vi "AFG3022_Arb_Fun_Control.vi"(10 "Channel":u16(ring) items=["Channel 1", "Channel 2"], 11 "Function Selector":u16(ring) items=["Sine", "Square", "Ramp", "Assymetric Sine", "Assymetric Arbitrary"]) -> ()   [LabVIEW 2012]
uses:
  ADAM Client/Sub VIs/ADAM Controls/Update_scan_value.ctl
panel:
  in  "Amp Gain":dbl=73.0
  in  "AM?":bool
  in  "Deviation Frequency":dbl=500.0
  in  "Modulation Frequency":dbl=20.0
  in  "FM?":bool
  in  "Channel 2 Phase":dbl
  in  "Channel 1 Phase":dbl
  in  "Set Zero Mean":bool
  out "Amplitude":dbl=120.0
  in  "Set Amplitude":bool
  out "Ts/T":dbl=0.32
  in  "Time Ratio":dbl[](array[slide])=[0.07, 0.15, 0.1, 0.6799999999999999] min=0.0 max=1.0 step=0.01 scale=0.0..1.0
  in  "Fine Amp":dbl(knob) min=0.0 max=1.0 step=0.1 scale=0.0..1.0
  in  "Course Amp":dbl(knob)=120.0 min=0.0 max=120.0 step=2.0 scale=0.0..120.0
  in  "Channel 2":bool
  in  "Channel 1":bool
  in  "Set Frequency":bool
  in  "Scale":u16(ring)=2 items=["1", "10", "100", "1k", "10k"]
  in  "Fine Freq":dbl(knob)=0.5 min=0.0 max=1.0 step=0.1 scale=0.0..1.0
  in  "Course Freq":dbl(knob)=9.0 min=0.0 max=10.0 step=1.0 scale=0.0..10.0
  in  "Stop Button":bool
  in  "VISA resource name":refnum<visa-resource-name>="USB0::0x0699::0x0347::C036837::INSTR"
  out "Frequency":dbl=950.0
  # "Suction Time"
  # "Blowing Time"
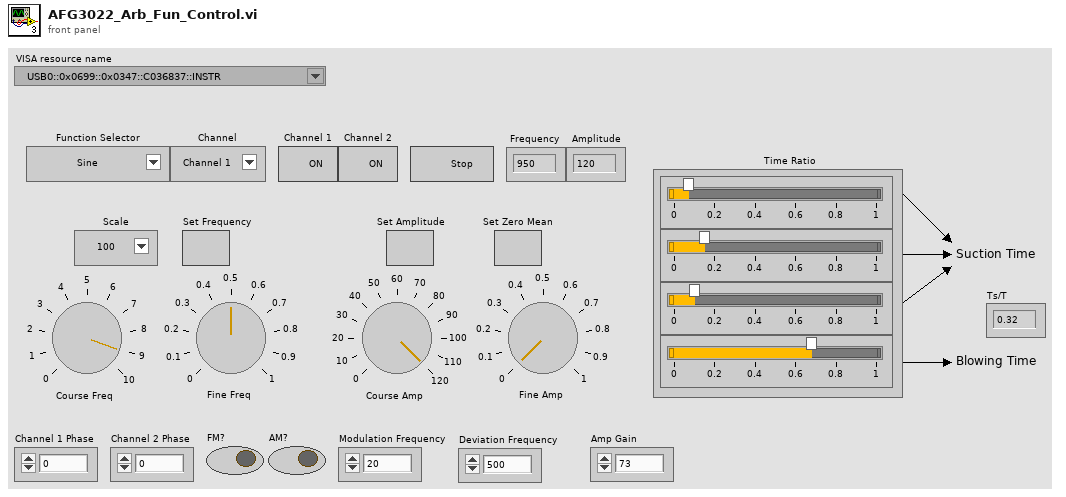
[diagram p1: front panel]
types:
  T1 = typedef "Update_scan_value.ctl" = cluster{"Channel Name":string, "New Value":dbl}
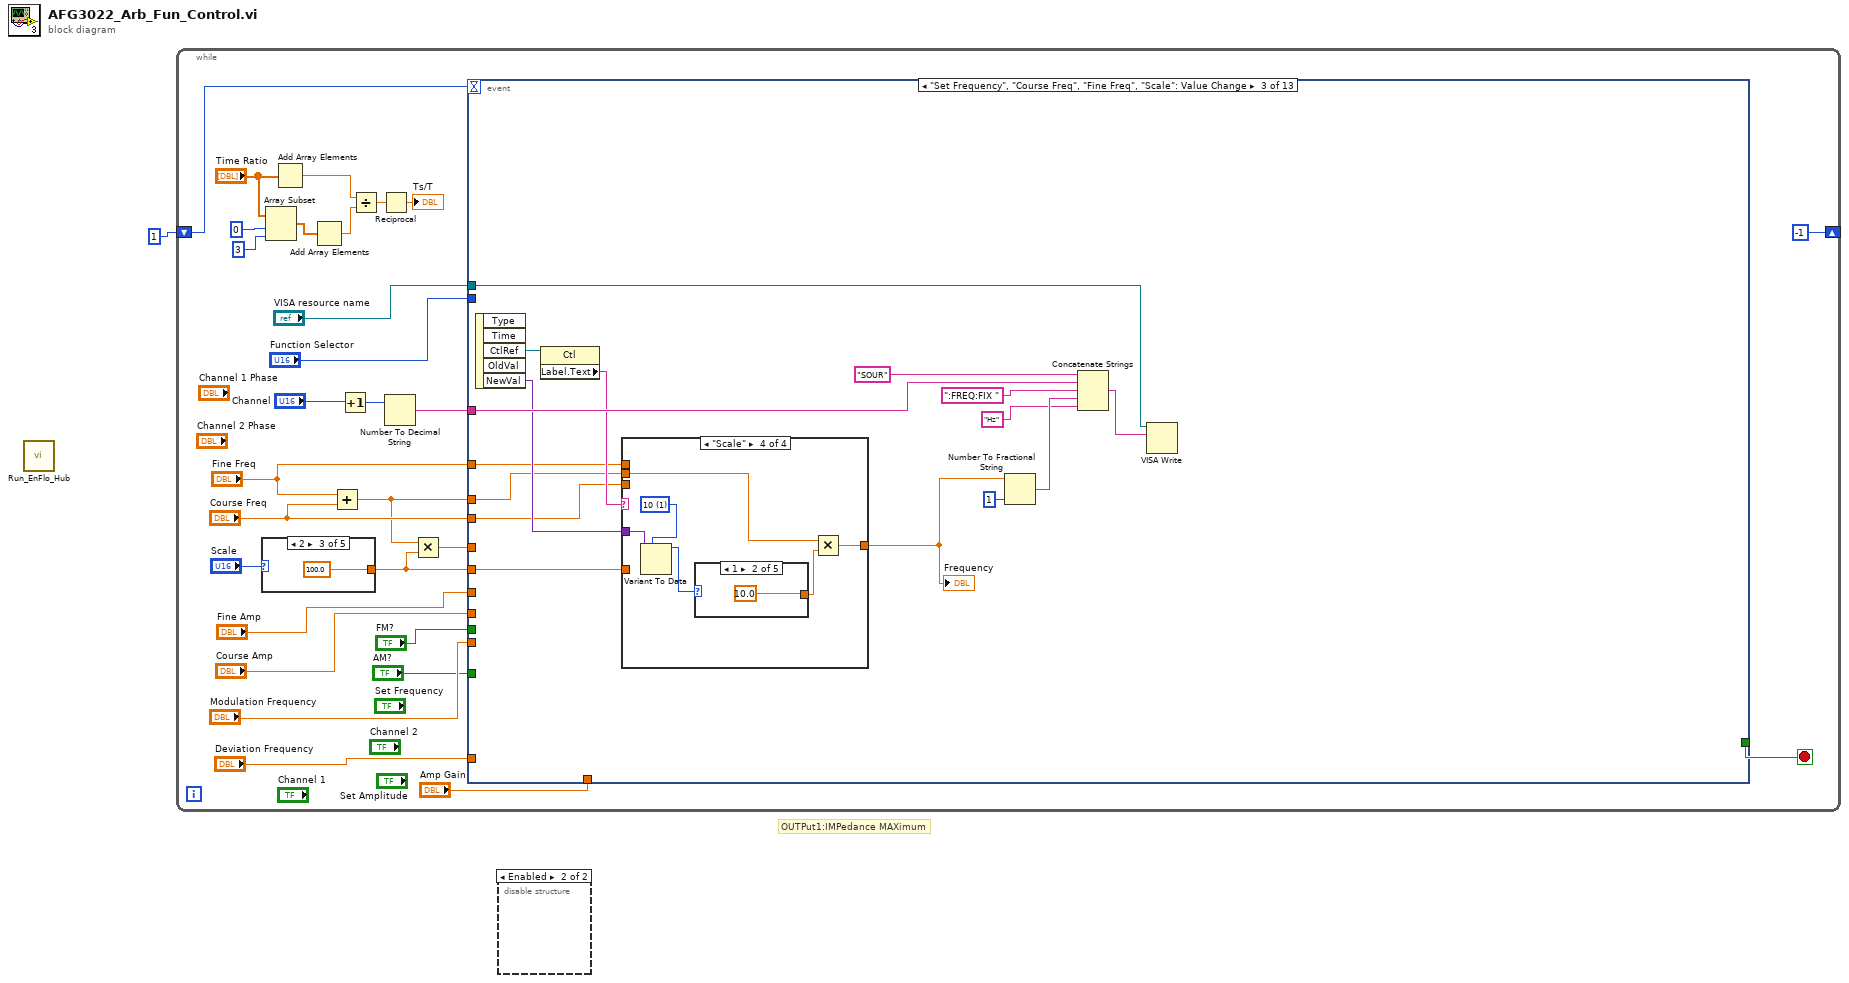
[diagram p0: block diagram]
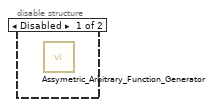
[diagram p2: hidden frame]
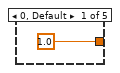
[diagram p3: hidden frame]
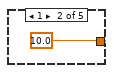
[diagram p4: hidden frame]
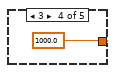
[diagram p5: hidden frame]
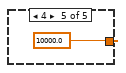
[diagram p6: hidden frame]
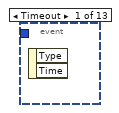
[diagram p7: hidden frame]
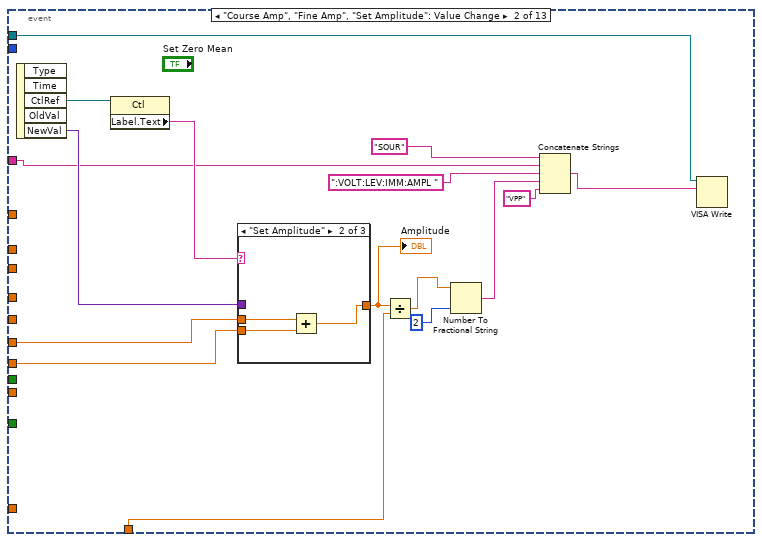
[diagram p8: hidden frame]
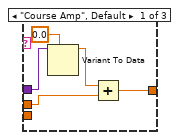
[diagram p9: hidden frame]
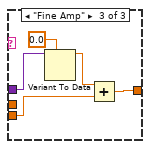
[diagram p10: hidden frame]
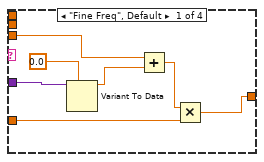
[diagram p11: hidden frame]
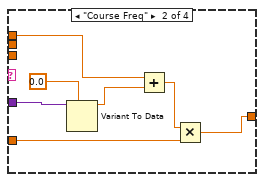
[diagram p12: hidden frame]
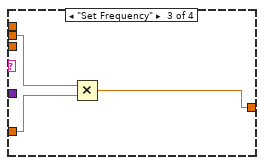
[diagram p13: hidden frame]
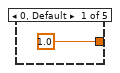
[diagram p14: hidden frame]
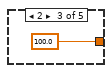
[diagram p15: hidden frame]
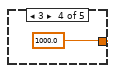
[diagram p16: hidden frame]
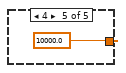
[diagram p17: hidden frame]
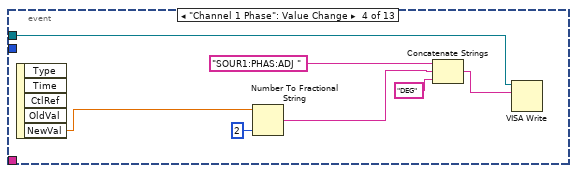
[diagram p18: hidden frame]
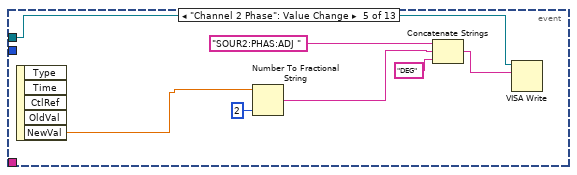
[diagram p19: hidden frame]
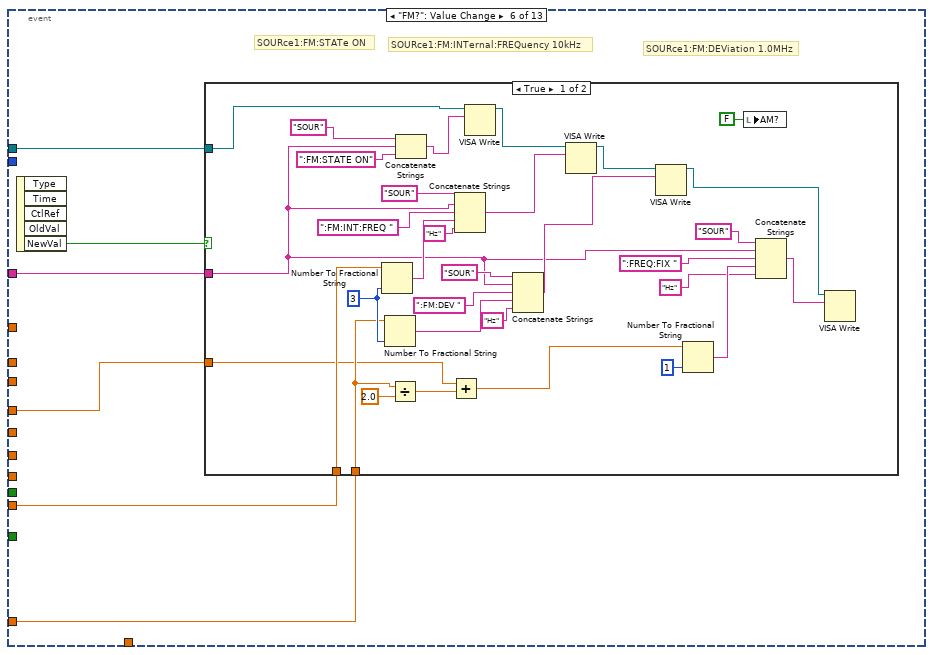
[diagram p20: hidden frame]
diagram:
  # "OUTPut1:IMPedance MAXimum"
  n1 = call "Run_EnFlo_Hub.vi"() -> ()  [unwired: 8 in]
  n2 = while {
    shift-right: [-1] -> _
    shift-left: 1 -> [w27]
    stop <- w29 stop-if-true
    n3 = case shown="2" "Scale" {
      tunnel: [1.0 10.0 100.0 1000.0 10000.0] -> w6
      frame 0, Default {
      }
      frame 1 {
      }
      frame 2 {
      }
      frame 3 {
      }
      frame 4 {
      }
    }
    n4 = Array Subset(array="Time Ratio", index=0, length=3) -> (w15:dbl[])
    n5 = Add Array Elements(numeric array="Time Ratio") -> (sum=w14:dbl)
    n6 = Add Array Elements(numeric array=w15) -> (sum=w13:dbl)
    n7 = Add(x="Fine Freq", y="Course Freq") -> (x+y=w5:dbl)
    n8 = Increment(x="Channel") -> (x+1=w25:u16)
    n9 = Divide(x=w14, y=w13) -> (x/y=w12:dbl)
    n10 = Reciprocal(x=w12) -> (1/x=→"Ts/T":dbl)
    n11 = Number To Decimal String(number=w25) -> (decimal integer string=w23:string)  [unwired: 1 in]
    n12 = Multiply(x=w5, y=w6) -> (x*y=w4:dbl)
    n13 = event shown="[2] \"Set Frequency\", \"Course Freq\", \"Fine Freq\", \"Scale\": Value Change" {
      selector: _ -> [_ _ _ _ _ _ _ _ _ _ _ _ _]
      dyn-events: _ -> [_ _ _ _ _ _ _ _ _ _ _ _ _]
      timeout: w27 -> [_ _ _ _ _ _ _ _ _ _ _ _ _]
      tunnel: "VISA resource name" -> [_ w39 w75 w113 w117 w126 w177 w220 w236 w265 w277 w309 _]
      tunnel: [_ _ _ _ _ _ _ _ _ _ _ _ "Stop Button"] -> w29
      tunnel: w23 -> [_ w40 w73 _ _ w127 w176 w219 w235 _ _ w288 _]
      tunnel: w5 -> [_ _ w69 _ _ _ _ _ _ _ _ _ _]
      tunnel: "Course Freq" -> [_ _ w67 _ _ _ _ _ _ _ _ _ _]
      tunnel: w6 -> [_ _ w66 _ _ _ _ _ _ _ _ _ _]
      tunnel: "Fine Freq" -> [_ _ w65 _ _ _ _ _ _ _ _ _ _]
      tunnel: "Course Amp" -> [_ w48 _ _ _ _ _ _ _ _ _ w289 _]
      tunnel: "Fine Amp" -> [_ w47 _ _ _ _ _ _ _ _ _ w290 _]
      tunnel: "Function Selector" -> [_ _ _ _ _ _ _ _ _ _ _ w286 _]
      tunnel: "Modulation Frequency" -> [_ _ _ _ _ w125 w175 _ _ _ _ _ _]
      tunnel: "FM?" -> [_ _ _ _ _ _ _ w215 w237 _ _ _ _]
      tunnel: "Deviation Frequency" -> [_ _ _ _ _ w124 _ _ _ _ _ _ _]
      tunnel: w4 -> [_ _ _ _ _ w123 w174 _ w233 _ _ _ _]
      tunnel: "AM?" -> [_ _ _ _ _ _ _ w217 _ _ _ _ _]
      tunnel: "Amp Gain" -> [_ w37 _ _ _ _ _ _ _ _ _ w282 _]
      event Timeout {
        n14 = event-data() -> ()  [unwired: 1 in, 2 out]
      }
      event "Course Amp", "Fine Amp", "Set Amplitude": Value Change {
        n15 = event-data() -> ("CtlRef"=w51:refnum<vi>, "NewVal"=w49:variant)  [unwired: 1 in, 3 out]
        n16 = property class="Ctl"(reference=w51) -> ("Label.Text"=w50:string)  [unwired: 1 in, 2 out]
        n17 = case shown="\"Set Amplitude\"" w50 {
          tunnel: w49 -> [w53 _ w61]
          tunnel: w48 -> [_ w58 w64]
          tunnel: w47 -> [w56 w59 _]
          tunnel: [w55 w57 w63] -> w36
          frame "Course Amp", Default {
            n18 = Variant To Data(type=0.0 ("Fine Amp"), Variant=w53) -> (data=w52:dbl)  [unwired: 1 in, 1 out]
            n19 = Add(x=w52, y=w56) -> (x+y=w55:dbl)
          }
          frame "Set Amplitude" {
            n20 = Add(x=w59, y=w58) -> (x+y=w57:dbl)
          }
          frame "Fine Amp" {
            n21 = Variant To Data(type=0.0 ("Fine Amp"), Variant=w61) -> (data=w60:dbl)  [unwired: 1 in, 1 out]
            n22 = Add(x=w60, y=w64) -> (x+y=w63:dbl)
          }
        }
        "Amplitude" <- w36
        n23 = Divide(x=w36, y=w37) -> (x/y=w38:dbl)
        n24 = Number To Fractional String(number=w38, precision (6)=i16 2) -> (F-format string=w42:string)  [unwired: 2 in]
        n25 = Concatenate Strings("SOUR" ("string"), w40, ":VOLT:LEV:IMM:AMPL " ("string"), w42, "VPP" ("string")) -> (w43:string)
        n26 = VISA Write(VISA resource name=w39, write buffer=w43) -> ()  [unwired: 1 in, 3 out]
      }
      event "Set Frequency", "Course Freq", "Fine Freq", "Scale": Value Change {
        n27 = event-data() -> ("CtlRef"=w72:refnum<vi>, "NewVal"=w70:variant)  [unwired: 1 in, 3 out]
        n28 = property class="Ctl"(reference=w72) -> ("Label.Text"=w71:string)  [unwired: 1 in, 2 out]
        n29 = case shown="\"Scale\"" w71 {
          tunnel: w70 -> [w87 w94 _ w103]
          tunnel: w69 -> [_ _ w97 w99]
          tunnel: [w81 w88 w95 w98] -> w68
          tunnel: w67 -> [w84 _ _ _]
          tunnel: w66 -> [w82 w90 w96 _]
          tunnel: w65 -> [_ w89 _ _]
          frame "Fine Freq", Default {
            n30 = Variant To Data(type=0.0, Variant=w87) -> (data=w85:dbl)  [unwired: 1 in, 1 out]
            n31 = Add(x=w84, y=w85) -> (x+y=w83:dbl)
            n32 = Multiply(x=w83, y=w82) -> (x*y=w81:dbl)
          }
          frame "Course Freq" {
            n33 = Variant To Data(type=0.0, Variant=w94) -> (data=w92:dbl)  [unwired: 1 in, 1 out]
            n34 = Add(x=w89, y=w92) -> (x+y=w91:dbl)
            n35 = Multiply(x=w91, y=w90) -> (x*y=w88:dbl)
          }
          frame "Set Frequency" {
            n36 = Multiply(x=w97, y=w96) -> (x*y=w95:dbl)
          }
          frame "Scale" {
            w102 = u16 1 items=["1", "10", "100", "1k", "10k"] ("Scale")
            n37 = Variant To Data(type=w102, Variant=w103) -> (data=w101:u16)  [unwired: 1 in, 1 out]
            n38 = case shown="1" w101 {
              tunnel: [1.0 10.0 100.0 1000.0 10000.0] -> w100
              frame 0, Default {
              }
              frame 1 {
              }
              frame 2 {
              }
              frame 3 {
              }
              frame 4 {
              }
            }
            n39 = Multiply(x=w99, y=w100) -> (x*y=w98:dbl)
          }
        }
        "Frequency" <- w68
        n40 = Number To Fractional String(number=w68, precision (6)=i16 1) -> (F-format string=w77:string)  [unwired: 2 in]
        n41 = Concatenate Strings("SOUR", w73, ":FREQ:FIX " ("string"), w77, "Hz" ("string")) -> (w74:string)
        n42 = VISA Write(VISA resource name=w75, write buffer=w74) -> ()  [unwired: 1 in, 3 out]
      }
      event "Channel 1 Phase": Value Change {
        n43 = event-data() -> ("NewVal"=w112:dbl)  [unwired: 1 in, 4 out]
        n44 = Number To Fractional String(number=w112, precision (6)=i16 2) -> (F-format string=w110:string)  [unwired: 2 in]
        n45 = Concatenate Strings("SOUR1:PHAS:ADJ ", w110, "DEG" ("string")) -> (w114:string)
        n46 = VISA Write(VISA resource name=w113, write buffer=w114) -> ()  [unwired: 1 in, 3 out]
      }
      event "Channel 2 Phase": Value Change {
        n47 = event-data() -> ("NewVal"=w116:dbl)  [unwired: 1 in, 4 out]
        n48 = Number To Fractional String(number=w116, precision (6)=i16 2) -> (F-format string=w119:string)  [unwired: 2 in]
        n49 = Concatenate Strings("SOUR2:PHAS:ADJ ", w119, "DEG" ("string")) -> (w121:string)
        n50 = VISA Write(VISA resource name=w117, write buffer=w121) -> ()  [unwired: 1 in, 3 out]
      }
      event "FM?": Value Change {
        # "SOURce1:FM:DEViation 1.0MHz"
        # "SOURce1:FM:INTernal:FREQuency 10kHz"
        # "SOURce1:FM:STATe ON"
        n51 = event-data() -> ("NewVal"=w128:bool)  [unwired: 1 in, 4 out]
        n52 = case shown="True" w128 {
          tunnel: w127 -> [w131 w162]
          tunnel: w126 -> [w158 w171]
          tunnel: w125 -> [w152 _]
          tunnel: w124 -> [w144 _]
          tunnel: w123 -> [w142 w161]
          frame True {
            w149 = i16 3 ("precision (6)")
            n53 = Number To Fractional String(number=w152, precision (6)=w149) -> (F-format string=w151:string)  [unwired: 2 in]
            n54 = Number To Fractional String(number=w144, precision (6)=w149) -> (F-format string=w146:string)  [unwired: 2 in]
            n55 = Divide(x=w144, y=2.0) -> (x/y=w141:dbl)
            n56 = Concatenate Strings("SOUR", w131, ":FM:STATE ON" ("string")) -> (w157:string)
            n57 = Add(x=w142, y=w141) -> (x+y=w130:dbl)
            n58 = Concatenate Strings("SOUR", w131, ":FM:INT:FREQ " ("string"), w151, "Hz" ("string")) -> (w153:string)
            n59 = VISA Write(VISA resource name=w158, write buffer=w157) -> (VISA resource name out=w156:refnum<visa-resource-name>)  [unwired: 1 in, 2 out]
            n60 = Concatenate Strings("SOUR", w131, ":FM:DEV " ("string"), w146, "Hz" ("string")) -> (w134:string)
            n61 = VISA Write(VISA resource name=w156, write buffer=w153) -> (VISA resource name out=w133:refnum<visa-resource-name>)  [unwired: 1 in, 2 out]
            n62 = VISA Write(VISA resource name=w133, write buffer=w134) -> (VISA resource name out=w132:refnum<visa-resource-name>)  [unwired: 1 in, 2 out]
            n63 = Number To Fractional String(number=w130, precision (6)=i16 1) -> (F-format string=w137:string)  [unwired: 2 in]
            n64 = local write "AM?"(FALSE ("AM?")) -> ()
            n65 = Concatenate Strings("SOUR", w131, ":FREQ:FIX " ("string"), w137, "Hz" ("string")) -> (w135:string)
            n66 = VISA Write(VISA resource name=w132, write buffer=w135) -> ()  [unwired: 1 in, 3 out]
          }
          frame False {
            n67 = Concatenate Strings("SOUR", w162, ":FM:STATE OFF" ("string")) -> (w170:string)
            n68 = VISA Write(VISA resource name=w171, write buffer=w170) -> (VISA resource name out=w163:refnum<visa-resource-name>)  [unwired: 1 in, 2 out]
            n69 = Number To Fractional String(number=w161, precision (6)=i16 1) -> (F-format string=w166:string)  [unwired: 2 in]
            n70 = Concatenate Strings("SOUR", w162, ":FREQ:FIX " ("string"), w166, "Hz" ("string")) -> (w164:string)
            n71 = VISA Write(VISA resource name=w163, write buffer=w164) -> ()  [unwired: 1 in, 3 out]
          }
        }
      }
      event "AM?": Value Change {
        n72 = event-data() -> ("NewVal"=w178:bool)  [unwired: 1 in, 4 out]
        n73 = case shown="True" w178 {
          tunnel: w177 -> [w180 w193]
          tunnel: w176 -> [w179 w209]
          tunnel: w175 -> [_ w200]
          tunnel: w174 -> [_ w185]
          frame False {
            # "SOURce1:AM:STATe OFF"
            n74 = Concatenate Strings("SOUR" ("string"), w179) -> (w181:string)
            n75 = Concatenate Strings(w181, ":AM:STAT OFF" ("string")) -> (w182:string)
            n76 = VISA Write(VISA resource name=w180, write buffer=w182) -> ()  [unwired: 1 in, 3 out]
          }
          frame True {
            # "SOURce1:AM:STATe OFF"
            # "SOURce1:AM:INTernal:FUNCtion SQUare"
            # "SOURce1:AM:INTernal:FREQuency XXHz"
            # "SOURce1:AM:DEPth 100"
            n77 = Number To Fractional String(number=w185, precision (6)=i16 3) -> (F-format string=w188:string)  [unwired: 2 in]
            n78 = Number To Fractional String(number=w200, precision (6)=i16 3) -> (F-format string=w197:string)  [unwired: 2 in]
            n79 = Concatenate Strings("SOUR" ("string"), w209) -> (w191:string)
            n80 = Concatenate Strings(w191, ":AM:INT:FREQ " ("string"), w197, "Hz" ("string")) -> (w199:string)
            n81 = Concatenate Strings(w191, ":AM:STAT ON" ("string")) -> (w207:string)
            n82 = Concatenate Strings(w191, ":AM:DEPT 100" ("string")) -> (w205:string)
            n83 = Concatenate Strings(w191, ":AM:INT:FUNC SQU" ("string")) -> (w194:string)
            n84 = Concatenate Strings(w191, ":FREQ:FIX " ("string"), w188, "Hz" ("string")) -> (w190:string)
            n85 = VISA Write(VISA resource name=w193, write buffer=w190) -> (VISA resource name out=w192:refnum<visa-resource-name>)  [unwired: 1 in, 2 out]
            n86 = VISA Write(VISA resource name=w192, write buffer=w207) -> (VISA resource name out=w211:refnum<visa-resource-name>, error out=w204:errorcluster)  [unwired: 1 in, 1 out]
            n87 = VISA Write(VISA resource name=w211, write buffer=w205, error in (no error)=w204) -> (VISA resource name out=w213:refnum<visa-resource-name>, error out=w203:errorcluster)  [unwired: 1 out]
            n88 = VISA Write(VISA resource name=w213, write buffer=w199, error in (no error)=w203) -> (VISA resource name out=w212:refnum<visa-resource-name>, error out=w202:errorcluster)  [unwired: 1 out]
            n89 = VISA Write(VISA resource name=w212, write buffer=w194, error in (no error)=w202) -> ()  [unwired: 3 out]
            n90 = local write "FM?"(FALSE ("AM?")) -> ()
          }
        }
      }
      event "Modulation Frequency": Value Change {
        n91 = event-data() -> ("NewVal"=w218:dbl)  [unwired: 1 in, 4 out]
        n92 = Or(x=w215, y=w217) -> (x .or. y?=w216:bool)
        n93 = case shown="True" w216 {
          tunnel: w220 -> [_ w225]
          tunnel: w219 -> [_ w224]
          tunnel: w218 -> [_ w223]
          tunnel: w215 -> [_ w221]
          frame False {
          }
          frame True {
            # ":AM:INT:FREQ"
            n94 = case shown="False" w221 {
              tunnel: [":AM:INT:FREQ " ("string") ":FM:INT:FREQ " ("string")] -> w229
              frame False {
              }
              frame True {
              }
            }
            n95 = Number To Fractional String(number=w223, precision (6)=i16 3) -> (F-format string=w227:string)  [unwired: 2 in]
            n96 = Concatenate Strings("SOUR", w224, w229, w227, "Hz" ("string")) -> (w222:string)
            n97 = VISA Write(VISA resource name=w225, write buffer=w222) -> ()  [unwired: 1 in, 3 out]
          }
        }
      }
      event "Deviation Frequency": Value Change {
        n98 = event-data() -> ("NewVal"=w234:dbl)  [unwired: 1 in, 4 out]
        n99 = case shown="True" w237 {
          tunnel: w236 -> [_ w243]
          tunnel: w235 -> [_ w241]
          tunnel: w234 -> [_ w239]
          tunnel: w233 -> [_ w238]
          frame False {
          }
          frame True {
            n100 = Number To Fractional String(number=w239, precision (6)=i16 3) -> (F-format string=w254:string)  [unwired: 2 in]
            n101 = Divide(x=w239, y=2.0) -> (x/y=w251:dbl)
            n102 = Add(x=w238, y=w251) -> (x+y=w244:dbl)
            n103 = Concatenate Strings("SOUR", w241, ":FM:DEV: " ("string"), w254, "Hz" ("string")) -> (w242:string)
            n104 = VISA Write(VISA resource name=w243, write buffer=w242) -> (VISA resource name out=w240:refnum<visa-resource-name>)  [unwired: 1 in, 2 out]
            n105 = Number To Fractional String(number=w244, precision (6)=i16 1) -> (F-format string=w247:string)  [unwired: 2 in]
            n106 = Concatenate Strings("SOUR", w241, ":FREQ:FIX " ("string"), w247, "Hz" ("string")) -> (w245:string)
            n107 = VISA Write(VISA resource name=w240, write buffer=w245) -> ()  [unwired: 1 in, 3 out]
          }
        }
      }
      event "Channel 1": Value Change {
        n108 = event-data() -> ("NewVal"=w260:bool)  [unwired: 1 in, 4 out]
        n109 = case shown="False" w260 {
          tunnel: w265 -> [w266 w269]
          frame False {
            n110 = VISA Write(VISA resource name=w266, write buffer="OUTP1:STAT OFF") -> ()  [unwired: 1 in, 3 out]
          }
          frame True {
            n111 = VISA Write(VISA resource name=w269, write buffer="OUTP1:STAT ON") -> ()  [unwired: 1 in, 3 out]
          }
        }
        n112 = Boolean To (0,1)(Boolean=w260) -> (0, 1=w259:i16)
        n113 = Bundle By Name(cluster=T1 {"Channel Name"="", "New Value"=0.0} ("Update Scan Value Cluster"), "Channel Name"="Synthetic_Jet:Channel1:State" ("write buffer"), "New Value"=w259) -> (w262:T1)
        n114 = Build Array(w262) -> (w263:T1[])
        n115 = call "Update_Current_Value_client.vi"("Don't Bother with check?"=TRUE, "Update array in"=w263) -> ()
      }
      event "Channel 2": Value Change {
        n116 = event-data() -> ("NewVal"=w271:bool)  [unwired: 1 in, 4 out]
        n117 = case shown="False" w271 {
          tunnel: w277 -> [w278 w280]
          frame False {
            n118 = VISA Write(VISA resource name=w278, write buffer="OUTP2:STAT OFF") -> ()  [unwired: 1 in, 3 out]
          }
          frame True {
            n119 = VISA Write(VISA resource name=w280, write buffer="OUTP2:STAT ON") -> ()  [unwired: 1 in, 3 out]
          }
        }
        n120 = Boolean To (0,1)(Boolean=w271) -> (0, 1=w272:i16)
        n121 = Bundle By Name(cluster=T1 {"Channel Name"="", "New Value"=0.0} ("Update Scan Value Cluster"), "Channel Name"="Synthetic_Jet:Channel2:State" ("write buffer"), "New Value"=w272) -> (w274:T1)
        n122 = Build Array(w274) -> (w275:T1[])
        n123 = call "Update_Current_Value_client.vi"("Don't Bother with check?"=TRUE, "Update array in"=w275) -> ()
      }
      event "Function Selector", "Time Ratio", "Set Zero Mean": Value Change {
        n124 = event-data() -> ("CtlRef"=w307:refnum<vi>, "OldVal"=w285:variant, "NewVal"=w305:variant)  [unwired: 1 in, 2 out]
        n125 = property class="Ctl"(reference=w307) -> ("Label.Text"=w306:string)  [unwired: 1 in, 2 out]
        n126 = Add(x=w290, y=w289) -> (x+y=w284:dbl)
        n127 = Divide(x=w284, y=w282) -> (x/y=w283:dbl)
        n128 = case shown="\"Set Zero Mean\"" w306 {
          tunnel: w305 -> [w317 w354 _]
          tunnel: [w316 w353 w356] -> w304
          tunnel: [w311 w352 w355] -> w303
          tunnel: w286 -> [w310 w351 w356]
          tunnel: w285 -> [w315 _ _]
          frame "Time Ratio" {
            w313 = dbl[] []
            n129 = Variant To Data(type=w313, Variant=w315) -> (data=w314:dbl[])  [unwired: 1 in, 1 out]
            n130 = Variant To Data(type=w313, Variant=w317) -> (data=w312:dbl[])  [unwired: 1 in, 1 out]
            n131 = case shown="3" w310 {
              selector: w310 -> [w318 w336]
              tunnel: [w318 w336] -> w316
              tunnel: w314 -> [w331 w350]
              tunnel: w312 -> [w322 w338]
              tunnel: [w319 w337] -> w311
              frame 4, Default {
                n132 = for {
                  tunnel: w331 -> [w335] mode=indexing
                  tunnel: w322 -> [w334] mode=indexing
                  tunnel: [w332] -> w330
                  i -> [w332]
                  stop <- w333 stop-if-true
                  n133 = Not Equal?(x=w335, y=w334) -> (x != y?=w333:bool)
                }
                n134 = Add Array Elements(numeric array=w322) -> (sum=w329:dbl)
                n135 = Decrement(x=w329) -> (x-1=w323:dbl)
                n136 = Equal?(x=3, y=w330) -> (x = y?=w327:bool)
                n137 = Select(t=1, s=w327, f=3 ("t")) -> (s? t:f=w320:i32)
                n138 = Index Array(array=w322, index=w320) -> (element=w324:dbl)
                n139 = Subtract(x=w324, y=w323) -> (x-y=w321:dbl)
                n140 = Replace Array Subset(array=w322, new element=w321, index=w320) -> (w319:dbl[])
                n141 = local write "Time Ratio"(w319) -> ()
              }
              frame 3 {
                w348 = 3 ("index")
                n142 = Index Array(array=w350, index=w348) -> (element=w349:dbl)
                n143 = Index Array(array=w338, index=w348) -> (element=w347:dbl)
                n144 = Not Equal?(x=w349, y=w347) -> (x != y?=w343:bool)
                n145 = Add Array Elements(numeric array=w338) -> (sum=w346:dbl)
                n146 = Decrement(x=w346) -> (x-1=w340:dbl)
                n147 = Select(t=1, s=w343, f=3 ("t")) -> (s? t:f=w342:i32)
                n148 = Index Array(array=w338, index=w342) -> (element=w341:dbl)
                n149 = Subtract(x=w341, y=w340) -> (x-y=w339:dbl)
                n150 = Replace Array Subset(array=w338, new element=w339, index=w342) -> (w337:dbl[])
                n151 = local write "Time Ratio"(w337) -> ()
              }
            }
          }
          frame "Function Selector", Default {
            n152 = Variant To Data(type=w351, Variant=w354) -> (data=w353:u16)  [unwired: 1 in, 1 out]
            n153 = local read "Time Ratio"() -> (w352:dbl[])
          }
          frame "Set Zero Mean" {
            n154 = local read "Time Ratio"() -> (w355:dbl[])
          }
        }
        n155 = Number To Fractional String(number=0.0, precision (6)=i16 4) -> (F-format string=w295:string)  [unwired: 2 in]
        n156 = Number To Fractional String(number=w283, precision (6)=i16 4) -> (F-format string=w300:string)  [unwired: 2 in]
        n157 = Concatenate Strings("SOUR" ("string"), w288, ":VOLT:LEV:IMM:OFFS " ("string")) -> (w296:string)
        n158 = Concatenate Strings(w296, w295, "V;:SOUR" ("string"), w288) -> (w298:string)
        n159 = Concatenate Strings(w298, ":VOLT:LEV:IMM:AMPL " ("string"), w300, "VPP" ("string")) -> (w287:string)
        n160 = case shown="100" w304 {
          tunnel: w309 -> [w364 w369 w375 w407 w434 _]
          tunnel: w288 -> [w359 w368 w377 w394 w424 _]
          tunnel: ":FUNC:SHAP " ("string") -> [w362 w367 w376 _ _ _]
          tunnel: w290 -> [_ _ _ w409 w436 _]
          tunnel: w289 -> [_ _ _ w408 w435 _]
          tunnel: w303 -> [_ _ _ w388 w414 _]
          tunnel: w287 -> [w357 w366 w373 _ _ _]
          tunnel: w282 -> [_ _ _ w382 w411 _]
          frame 0, Default {
            n161 = Concatenate Strings("SOUR" ("string"), w359, w362, "SIN" ("string")) -> (w360:string)
            n162 = VISA Write(VISA resource name=w364, write buffer=w360) -> (VISA resource name out=w358:refnum<visa-resource-name>)  [unwired: 1 in, 2 out]
            n163 = VISA Write(VISA resource name=w358, write buffer=w357) -> ()  [unwired: 1 in, 3 out]
          }
          frame 1 {
            n164 = Concatenate Strings("SOUR" ("string"), w368, w367, "SQU" ("string")) -> (w370:string)
            n165 = VISA Write(VISA resource name=w369, write buffer=w370) -> (VISA resource name out=w365:refnum<visa-resource-name>)  [unwired: 1 in, 2 out]
            n166 = VISA Write(VISA resource name=w365, write buffer=w366) -> ()  [unwired: 1 in, 3 out]
          }
          frame 2 {
            n167 = Concatenate Strings("SOUR" ("string"), w377, w376, "RAMP" ("string")) -> (w378:string)
            n168 = VISA Write(VISA resource name=w375, write buffer=w378) -> (VISA resource name out=w374:refnum<visa-resource-name>)  [unwired: 1 in, 2 out]
            n169 = VISA Write(VISA resource name=w374, write buffer=w373) -> ()  [unwired: 1 in, 3 out]
          }
          frame 3 {
            n170 = Add(x=w409, y=w408) -> (x+y=w383:dbl)
            n171 = Index Array(array=w388, index=3) -> (element=w387:dbl)
            n172 = Divide(x=w383, y=w382) -> (x/y=w381:dbl)
            n173 = Subtract(x=1.0, y=w387) -> (x-y=w385:dbl)
            n174 = Concatenate Strings("SOUR" ("string"), w394, ":VOLT:LEV:IMM:OFFS " ("string")) -> (w397:string)
            n175 = call "Assymetric_Sine_Wave.vi"("Ts"=w385, "Ub"=w381, "samples"=1000) -> ("offset"=w395:dbl, "amplitude"=w403:dbl, "Assymetric Sign Wave"=w406:dbl[])  [unwired: 6 in]
            n176 = Number To Fractional String(number=w395, precision (6)=i16 4) -> (F-format string=w398:string)  [unwired: 2 in]
            n177 = Number To Fractional String(number=w403, precision (6)=i16 4) -> (F-format string=w391:string)  [unwired: 2 in]
            n178 = call "Transfer_Arb_Waveform.vi"("Channel"=w394, "Arbitrary Waveform"=w406, "VISA resource name"=w407) -> ("error out"=w404:errorcluster, "VISA resource name out"=w405:refnum<visa-resource-name>)  [unwired: 7 in]
            n179 = Concatenate Strings(w397, w398, "V;:SOUR" ("string"), w394) -> (w393:string)
            n180 = Concatenate Strings(w393, ":VOLT:LEV:IMM:AMPL " ("string"), w391, "VPP" ("string")) -> (w389:string)
            n181 = VISA Write(VISA resource name=w405, write buffer=w389, error in (no error)=w404) -> ()  [unwired: 3 out]
          }
          frame 4 {
            n182 = Add(x=w436, y=w435) -> (x+y=w413:dbl)
            n183 = Divide(x=w413, y=w411) -> (x/y=w412:dbl)
            n184 = Concatenate Strings("SOUR" ("string"), w424, ":VOLT:LEV:IMM:OFFS " ("string")) -> (w426:string)
            n185 = call "Assymetric_Arbitrary_Wave.vi"("Time Ratios"=w414, "Ub"=w412, "samples"=1000) -> ("offset"=w416:dbl, "amplitude"=w417:dbl, "Arbitary Assymetric Waveform"=w418:dbl[])  [unwired: 6 in]
            n186 = Number To Fractional String(number=w416, precision (6)=i16 4) -> (F-format string=w427:string)  [unwired: 2 in]
            n187 = Number To Fractional String(number=w417, precision (6)=i16 4) -> (F-format string=w421:string)  [unwired: 2 in]
            n188 = call "Transfer_Arb_Waveform.vi"("Channel"=w424, "Arbitrary Waveform"=w418, "VISA resource name"=w434) -> ("error out"=w432:errorcluster, "VISA resource name out"=w433:refnum<visa-resource-name>)  [unwired: 7 in]
            n189 = Concatenate Strings(w426, w427, "V;:SOUR" ("string"), w424) -> (w423:string)
            n190 = Concatenate Strings(w423, ":VOLT:LEV:IMM:AMPL " ("string"), w421, "VPP" ("string")) -> (w419:string)
            n191 = VISA Write(VISA resource name=w433, write buffer=w419, error in (no error)=w432) -> ()  [unwired: 3 out]
          }
          frame 100 {
          }
        }
      }
      event "Stop Button": Value Change {
        n192 = event-data() -> ()  [unwired: 1 in, 5 out]
      }
    }
  }
  n193 = disable-structure shown="Enabled" {
    frame Disabled {
      n194 = call "Assymetric_Arbitrary_Function_Generator.vi"() -> ()  [unwired: 9 in, 3 out]
    }
    frame Enabled {
    }
  }
